vi "Get Bag.vi"(8 "error in (no error)":errorcluster, 11 "Game in":refnum<class "Game.lvclass">) -> (0 "error out":errorcluster, 2 "Bag":refnum<class "Bag.lvclass">, 3 "Game out":refnum<class "Game.lvclass">)   [LabVIEW 2020, in "Game.lvclass"]
uses:
  Game.lvclass
  Bag/Bag.lvclass
  Game.lvclass/Game.ctl
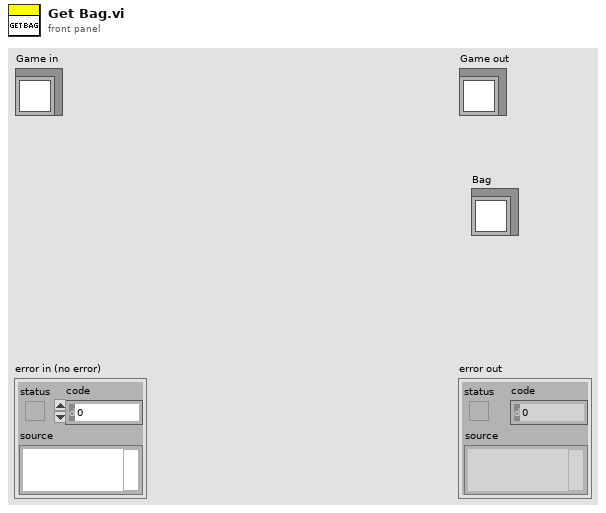
[diagram p1: front panel]
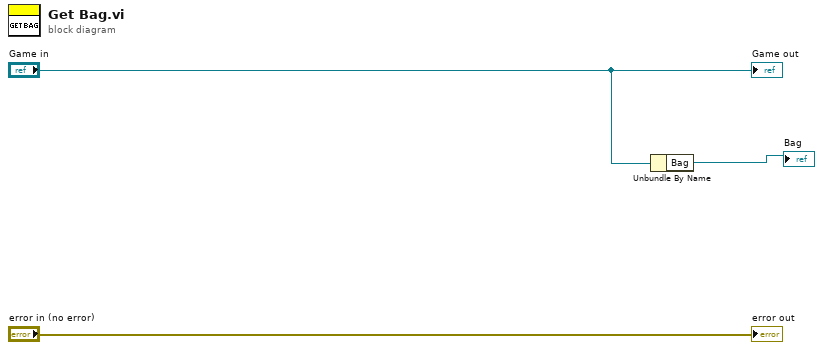
[diagram p0: block diagram]
diagram:
  n1 = Unbundle By Name("Game in") -> ("Bag"=→"Bag":refnum<class "Bag.lvclass">)
  "error out" <- "error in (no error)"
  "Game out" <- "Game in"
